vi "读取IO编译.vi"(11 "Read data":u8[](array[numeric])) -> (3 "Write Data":bool[](array[boolean]))   [LabVIEW 2014]
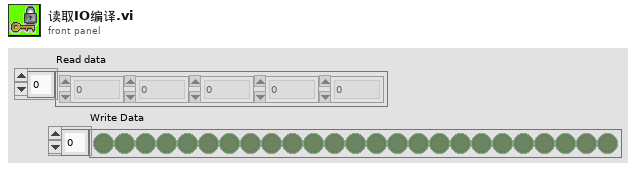
[diagram p1: front panel]
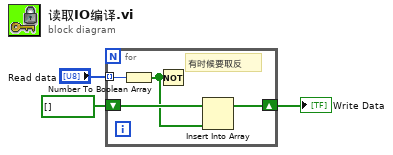
[diagram p0: block diagram]
diagram:
  n1 = for {
    tunnel: "Read data" -> [w7] mode=indexing
    shift-right: [w5] -> w1
    shift-left: bool[] [] -> [w6]
    # "有时候要取反"
    n2 = Number To Boolean Array(number=w7) -> (Boolean array=w4:bool[])
    n3 = Not(x=w4) -> ()  [unwired: 1 out]
    n4 = Insert Into Array(array=w6, new element=w4) -> (w5:bool[])  [unwired: 1 in]
  }
  "Write Data" <- w1
